vi "Get Sensitivity.vi"(6 "sensitivity":sgl, 7 "pa":i32, 8 "error in (no error)":errorcluster, 9 "amplifier":i32, 10 "horzShift":i32, 11 "channel":i32) -> (0 "error out":errorcluster, 3 "function return":u32, 4 "sensitivity out":sgl)   [LabVIEW 2014, in "atmcd32d.lvlib"]
doc: "unsigned int WINAPI GetSensitivity(int channel, int horzShift, int amplifier, int pa, float * sensitivity);"
uses:
  atmcd32d.lvlib
  atmcd32d.dll
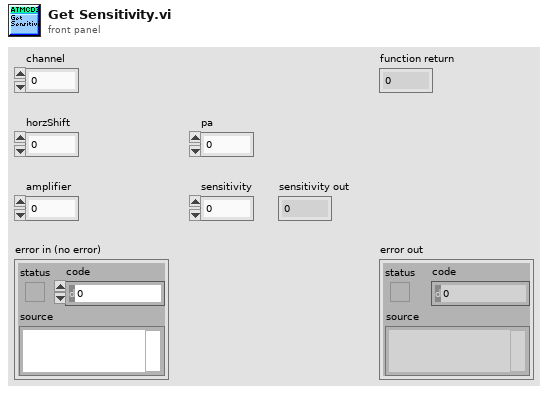
[diagram p1: front panel]
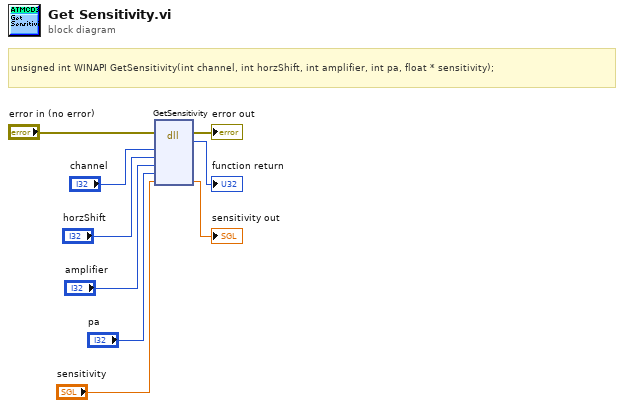
[diagram p0: block diagram]
diagram:
  # "unsigned int WINAPI GetSensitivity(int channel, int horzShift, int amplifier, int pa, float * sensitivity);"
  n1 = dll-call lib="C:/Users/Bakir/Documents/Lambda2-Testing/lib/Andorlib/atmcd32d.*" fn="GetSensitivity"(error in="error in (no error)", "channel"="channel", "horzShift"="horzShift", "amplifier"="amplifier", "pa"="pa", "sensitivity"="sensitivity") -> (error out=→"error out":errorcluster, →"function return":u32, "sensitivity"=→"sensitivity out":sgl)  [unwired: 6 in, 1 out]
